vi "ESP301 Status.vi"(5 "Axe Inv":bool, 6 "Input Units":i8(ring) items=["mm", "ps"], 7 "ESP301Ref":T1, 8 "error in":errorcluster, 9 "Axis":i8(ring)=1 items=["Axis 1"=1, "Axis 2"=2, "Axis 3"=3], 11 "VISA Rsrc":refnum<visa-resource-name>="GPIB0::7::INSTR") -> (0 "error out":errorcluster, 1 "Position":dbl=0.5, 2 "Low Limit":bool[](array[boolean]), 3 "High Limit":bool[](array[boolean]))   [LabVIEW 2019]
uses:
  <userlib>/ESP300/ESP300 GotoState.ctl
  <userlib>/GenProg/WritebyRefNum.vi
panel:
  out "Status Reg1":bool[](array[boolean])
  out "Status Reg2":bool[](array[boolean])
  # "b2"
  # "1+"
  # "2-"
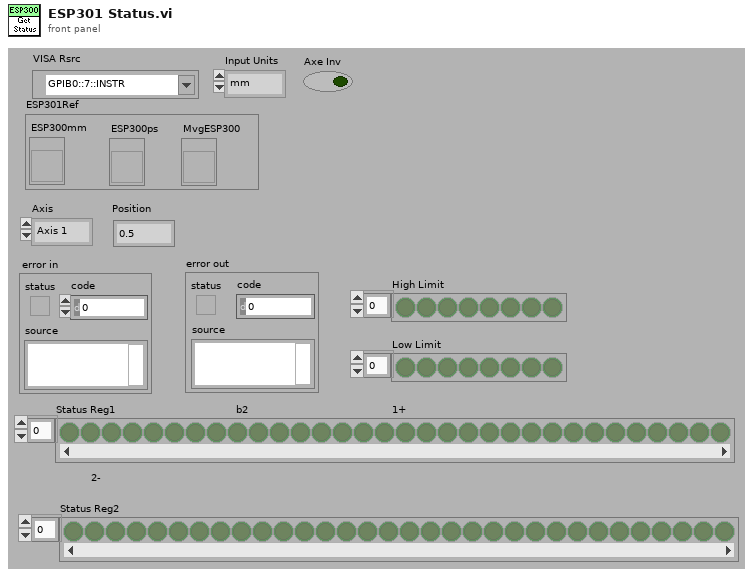
[diagram p1: front panel]
types:
  T1 = cluster{"ESP300mm":refnum<vi>, "ESP300ps":refnum<vi>, "MvgESP300":refnum<vi>}
  T2 = typedef "ESP300 GotoState.ctl" = enum16{"send command", "read position", "check status", "end"}
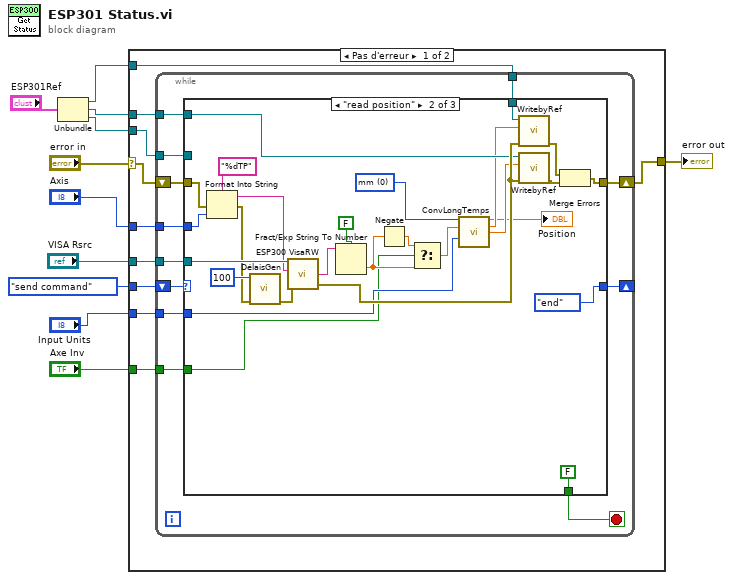
[diagram p0: block diagram]
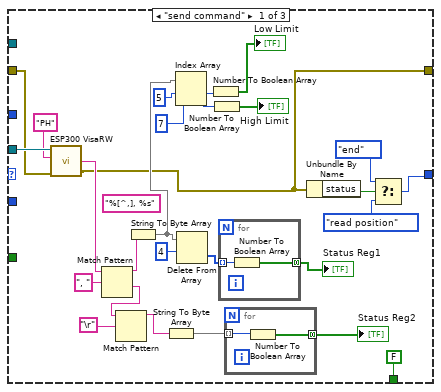
[diagram p2: hidden frame]
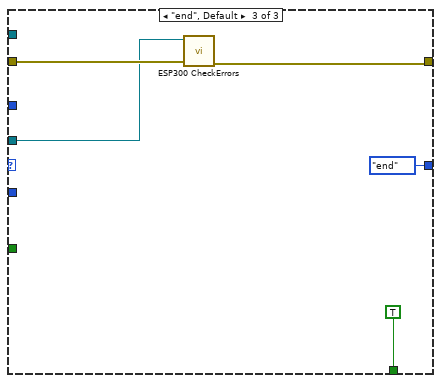
[diagram p3: hidden frame]
diagram:
  n1 = Unbundle("ESP301Ref") -> ("ESP300mm"=w2:refnum<vi>, "ESP300ps"=w4:refnum<vi>, "MvgESP300"=w3:refnum<vi>)
  n2 = case shown="Pas d'erreur" "error in" {
    selector: "error in" -> [w19 w97]
    tunnel: "Axis" -> [w21 _]
    tunnel: [w18 w97] -> w9
    tunnel: ESP300_GotoState."send command" ("Énum") -> [w20 _]
    tunnel: "VISA Rsrc" -> [w17 _]
    tunnel: w3 -> [w16 _]
    tunnel: "Input Units" -> [w15 _]
    tunnel: w2 -> [w14 _]
    tunnel: w4 -> [w13 _]
    tunnel: "Axe Inv" -> [w12 _]
    frame No Error {
      n3 = while {
        tunnel: w21 -> [w33]
        shift-right: [w29] -> w18
        shift-left: w19 -> [w31]
        tunnel: w17 -> [w30]
        shift-right: [w27] -> _
        shift-left: w20 -> [w32]
        tunnel: w16 -> [w26]
        tunnel: w15 -> [w25]
        tunnel: w14 -> [w24]
        tunnel: w13 -> [w23]
        tunnel: w12 -> [w22]
        stop <- w28 stop-if-true
        n4 = case shown="\"read position\"" w32 {
          tunnel: w33 -> [_ w89 _]
          tunnel: w31 -> [w54 w88 w94]
          tunnel: w30 -> [w60 w91 w92]
          tunnel: [w34 w79 w93] -> w29
          tunnel: [FALSE FALSE TRUE] -> w28
          tunnel: [w56 ESP300_GotoState."end" ("Énum") ESP300_GotoState."end" ("Énum")] -> w27
          tunnel: w26 -> [_ _ _]
          tunnel: w25 -> [_ w72 _]
          tunnel: w24 -> [_ w77 _]
          tunnel: w23 -> [_ w76 _]
          tunnel: w22 -> [_ w68 _]
          frame "send command" {
            (unwired) "%[^,], %s" ("chaîne de format")
            n5 = call <userlib>:"ESP300 VisaRW.vi"("error in (no error)"=w54, "ChaineCom"="PH" ("format string"), "VISA Rsrc"=w60) -> ("error out"=w34:errorcluster, "ChaineRep"=w50:string)  [unwired: 4 in, 2 out]
            n6 = Match Pattern(string=w50, regular expression=", " ("expression régulière")) -> (before substring=w48:string, after substring=w46:string)  [unwired: 1 in, 2 out]
            n7 = Match Pattern(string=w46, regular expression="\r") -> (before substring=w47:string)  [unwired: 1 in, 3 out]
            n8 = String To Byte Array(string=w48) -> (unsigned byte array=w41:u8[])
            n9 = String To Byte Array(string=w47) -> (unsigned byte array=w52:u8[])
            n10 = Index Array(array=w41, index #1=5 ("longueur"), index #2=7 ("longueur")) -> (element #1=w37:u8, element #2=w36:u8)
            n11 = Delete From Array(array=w41, length=4 ("longueur")) -> (deleted portion=w42:u8[])  [unwired: 1 in, 1 out]
            n12 = Number To Boolean Array(number=w37) -> (Boolean array=→"Low Limit":bool[])
            n13 = Number To Boolean Array(number=w36) -> (Boolean array=→"High Limit":bool[])
            n14 = for {
              tunnel: w42 -> [w64] mode=indexing
              tunnel: [w63] -> w51 mode=concatenating
              n15 = Number To Boolean Array(number=w64) -> (Boolean array=w63:bool[])
            }
            "Status Reg1" <- w51
            n16 = for {
              tunnel: w52 -> [w62] mode=indexing
              tunnel: [w61] -> w44 mode=concatenating
              n17 = Number To Boolean Array(number=w62) -> (Boolean array=w61:bool[])
            }
            "Status Reg2" <- w44
            n18 = Unbundle By Name(w34) -> ("status"=w58:bool)
            n19 = Select(t=ESP300_GotoState."end" ("Énum"), s=w58, f=ESP300_GotoState."read position" ("Énum")) -> (s? t:f=w56:T2)
          }
          frame "read position" {
            w75 = i8 0 items=["mm", "ps"] ("Input Units")
            n20 = Format Into String(format string="%dTP", error in=w88, w89) -> (resulting string=w87:string, error out=w82:errorcluster)  [unwired: 1 in]
            n21 = call "DélaisGen.vi"("error in (no error)"=w82, "ms To Wait"=u32 100 ("milliseconds to wait")) -> ("error out"=w83:errorcluster)  [unwired: 9 in]
            n22 = call <userlib>:"ESP300 VisaRW.vi"("error in (no error)"=w83, "ChaineCom"=w87, "VISA Rsrc"=w91) -> ("error out"=w80:errorcluster, "ChaineRep"=w86:string)  [unwired: 4 in, 2 out]
            n23 = Fract/Exp String To Number(use system decimal point (T)=FALSE ("utiliser le séparateur décimal du système (V)"), string=w86) -> (number=w70:dbl)  [unwired: 2 in, 1 out]
            n24 = Negate(x=w70) -> (-x=w71:dbl)
            n25 = Select(t=w71, s=w68, f=w70) -> (s? t:f=w69:dbl)
            n26 = call <userlib>:"ConvLongTemps.vi"("Input Units"=w75, "Units Input"=w69, "Output Units"=w72) -> ("Units Output"=→"Position":dbl, "Units mm"=w74:dbl, "Units ps"=w73:dbl)  [unwired: 9 in, 1 out]
            n27 = call-poly <userlib>:"WritebyRef.vi"("error in"=w80, "Valeur"=w74, "Control Ref"=w77) -> ("error out"=w78:errorcluster)  [unwired: 8 in]
            n28 = call-poly <userlib>:"WritebyRef.vi"("error in"=w80, "Valeur"=w73, "Control Ref"=w76) -> ("error out"=w81:errorcluster)  [unwired: 8 in]
            n29 = Merge Errors(w78, w81) -> (w79:errorcluster)
          }
          frame "end", Default {
            n30 = call <userlib>:"ESP300 CheckErrors.vi"("error in (no error)"=w94, "Ressource VISA In"=w92) -> ("error out"=w93:errorcluster)  [unwired: 4 in, 3 out]
          }
        }
      }
    }
    frame Error {
    }
  }
  "error out" <- w9
